vi "DIAdem Init.vi"(8 "error in (no error)":errorcluster, 10 "Startup DIAdem? (f)":bool) -> (0 "error out":errorcluster, 2 "Queues":T1, 3 "DIAdem Reference":T2)   [LabVIEW 2011]
uses:
  <vilib>/ExportToExcel/DIAdem Reference.ctl
  DIAdem Queues.ctl
  DIAdem Daemon Queue.ctl
  DIAdem Daemon Script Type.ctl
  Datasheet/Datasheet Inputs.ctl
  www/cgi-bin/_cgi-lib/TDM_INDEX Record.ctl
  Datasheet/Datasheet Generator Settings.ctl
  www/cgi-bin/runtest/runtest Queue.ctl
  www/tests/Test Output.ctl
  database/Fields/Field Record.ctl
  database/Fields/Field DataTypes.ctl
  database/Fields/Field NextItem.ctl
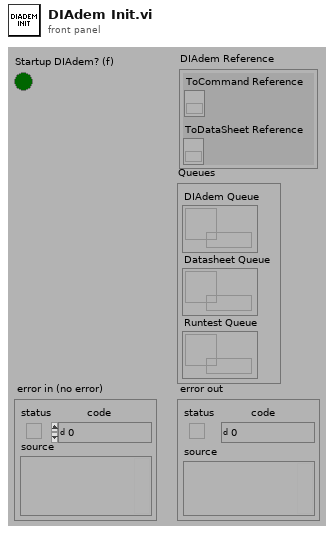
[diagram p1: front panel]
types:
  T1 = typedef "DIAdem Queues.ctl" = cluster{"DIAdem Queue":refnum<queue>, "Datasheet Queue":refnum<queue>, "Runtest Queue":refnum<queue>}
  T2 = typedef "DIAdem Reference.ctl" = cluster{"ToCommand Reference":refnum<k7>, "ToDataSheet Reference":refnum<k7>}
  T3 = typedef "runtest Queue.ctl" = cluster{"Test Output":T4, "Overwrite Existing?":bool, "Print?":bool, "sTestId":string, "Test Station IP (\"\")":string, "sxUsername (\"\")":string, "sDatasheetsCSV (\"\")":string, "Fields":T5[]}
  T4 = typedef "Test Output.ctl" = cluster{"Status":string, "Message":string, "Results":string, "Abort All":bool, "Save Results?":bool, "Timing Metrics":string}
  T5 = typedef "Field Record.ctl" = cluster{"ixField":i32, "iSequenceOrder":i32, "sxFieldId":string, "sxSequenceId":string, "sDisplayName":string, "sValue":string, "sUnits":string, "nDataType":T6, "nNextItem":T7, "fSystem":bool, "fSystemValue":bool, "fRequired":bool, "fSetAtTest":bool, "fTestField":bool, "fDeleted":bool, "fIndexed":bool, "fFreeList":bool}
  T6 = typedef "Field DataTypes.ctl" = enum32{"text", "numeric", "list", "timestamp", "boolean"}
  T7 = typedef "Field NextItem.ctl" = enum32{"Reset", "Retain", "Auto-Increment"}
  T8 = typedef "DATASHEET INPUTS.ctl" = cluster{"Items":T9[], "Templates":string[], "Generator Settings":T10, "Response Queue Name":string}
  T9 = typedef "TDM_INDEX Record.ctl" = cluster{"Model Number":string, "SN for sort":i32, "Test Type":string, "Test Run":string, "Serial Number":string, "Start Timestamp":timestamp, "Data File":path, "Result Columns":string[]}
  T10 = typedef "DATASHEET Generator Settings.ctl" = cluster{"Wait? (t)":bool, "ClientPrint? (f)":bool, "Client (\"\")":string, "joinPDF":bool, "Sort Method":enum16{"Item", "Template", "No Sort"}, "Export Row (-1=all)":i32, "Preview":bool, "Estimate Time":bool, "username":string, "jobid":string}
  T11 = typedef "DIAdem Daemon Queue.ctl" = cluster{"Report Template TDM":path, "Report Processor VBS":path, "Report Path PDF":path, "Report Script Params":string, "Username":string, "Script Type":T12, "Report Query Params":string, "Client Machine":string, "Print on Client?":bool, "Response Queue Name":string, "Script Variables":string[], "Start Request Time":timestamp, "Wait?":bool}
  T12 = typedef "DIAdem Daemon Script Type.ctl" = enum16{"Report", "Query", "Script", "Datasheet", "Append", "Restart", "Stop"}
  T13 = enum32{"invalid app kind", "Development System", "Run Time System", "Student Edition", "Embedded LabVIEW", "Evaluation", "Custom"}
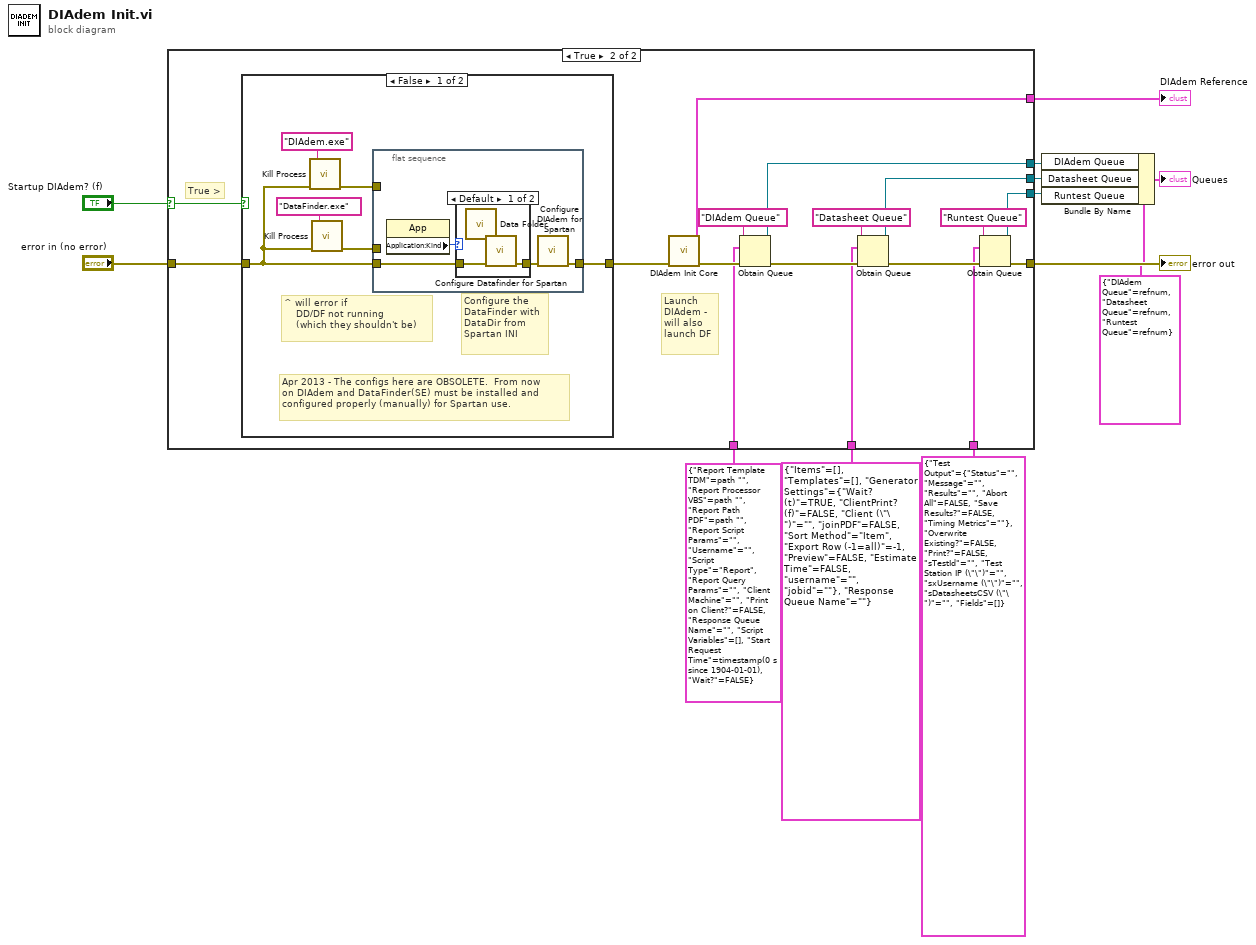
[diagram p0: block diagram]
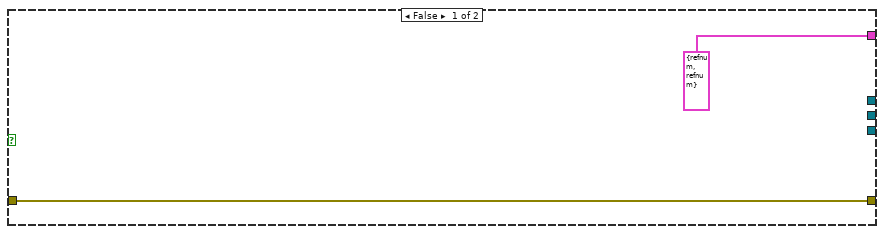
[diagram p2: hidden frame]
diagram:
  n1 = case shown="True" "Startup DIAdem? (f)" {
    selector: "Startup DIAdem? (f)" -> [_ w15]
    tunnel: "error in (no error)" -> [w14 w26]
    tunnel: [w14 w20] -> w11
    tunnel: [T2 {"ToCommand Reference"=refnum, "ToDataSheet Reference"=refnum} ("DIAdem Reference") w31] -> w9
    tunnel: [_ w28] -> w7
    tunnel: T11 {"Report Template TDM"=path "", "Report Processor VBS"=path "", "Report Path PDF"=path "", "Report Script Params"="", "Username"="", "Script Type"=enum."Report", "Report Query Params"="", "Client Machine"="", "Print on Client?"=FALSE, "Response Queue Name"="", "Script Variables"=[], "Start Request Time"=timestamp(0 s since 1904-01-01), "Wait?"=FALSE} ("DD_Report") -> [_ w25]
    tunnel: [_ w19] -> w6
    tunnel: [_ w18] -> w5
    tunnel: T8 {"Items"=[], "Templates"=[], "Generator Settings"={"Wait? (t)"=TRUE, "ClientPrint? (f)"=FALSE, "Client (\"\")"="", "joinPDF"=FALSE, "Sort Method"=enum."Item", "Export Row (-1=all)"=-1, "Preview"=FALSE, "Estimate Time"=FALSE, "username"="", "jobid"=""}, "Response Queue Name"=""} ("Datasheet Inputs") -> [_ w17]
    tunnel: T3 {"Test Output"={"Status"="", "Message"="", "Results"="", "Abort All"=FALSE, "Save Results?"=FALSE, "Timing Metrics"=""}, "Overwrite Existing?"=FALSE, "Print?"=FALSE, "sTestId"="", "Test Station IP (\"\")"="", "sxUsername (\"\")"="", "sDatasheetsCSV (\"\")"="", "Fields"=[]} ("INPUTS") -> [_ w16]
    frame False {
    }
    frame True {
      # "True >"
      # "Launch\nDIAdem -\nwill also\nlaunch DF"
      n2 = case shown="False" w15 {
        tunnel: [w36 w46] -> w27
        tunnel: w26 -> [w33 w46]
        frame False {
          # "Apr 2013 - The configs here are OBSOLETE.  From now\non DIAdem and DataFinder(SE) must be installed and\nconfigured properly (manually) for Spartan use."
          # "Configure the\nDataFinder with\nDataDir from\nSpartan INI"
          # "^ will error if\n    DD/DF not running\n    (which they shouldn't be)"
          n3 = call "Kill Process.vi"("error in (no error)"=w33, "Name of Process to kill (\"\")"="DIAdem.exe" ("Name of Process to kill (\"\")")) -> ("error out"=w32:errorcluster)  [unwired: 5 out]
          n4 = call "Kill Process.vi"("error in (no error)"=w33, "Name of Process to kill (\"\")"="DataFinder.exe" ("Name of Process to kill (\"\")")) -> ("error out"=w35:errorcluster)  [unwired: 5 out]
          n5 = flat-sequence {
            tunnel: w33 -> [w41]
            tunnel: [w39] -> w36
            tunnel: w35 -> [_]
            tunnel: w32 -> [_]
            frame #0 {
              n6 = property class="App"() -> ("Application:Kind"=w40:T13)  [unwired: 2 in, 2 out]
              n7 = case shown="Default" w40 {
                tunnel: w41 -> [w44 w45]
                tunnel: [w42 w45] -> w38
                frame Default {
                  n8 = call "Data Folder.vi"() -> ("Data Folder"=w43:path)  [unwired: 3 in]
                  n9 = call "Configure Datafinder for Spartan.vi"("error in (no error)"=w44, "Data Path"=w43) -> ("error out"=w42:errorcluster)  [unwired: 9 in]
                }
                frame "Development System" {
                }
              }
              n10 = call "Configure DIAdem for Spartan.vi"("error in (no error)"=w38) -> ("error out"=w39:errorcluster)  [unwired: 10 in]
            }
          }
        }
        frame True {
          # "This case should run - the FALSE case\nis there for reference."
        }
      }
      n11 = call "DIAdem Init Core.vi"("error in"=w27) -> ("error out"=w29:errorcluster, "DIAdem Reference"=w31:T2)  [unwired: 9 out]
      n12 = Obtain Queue(name (unnamed)="DIAdem Queue", element data type=w25, error in (no error)=w29) -> (queue out=w28:refnum<queue>, error out=w22:errorcluster)  [unwired: 2 in, 1 out]
      n13 = Obtain Queue(name (unnamed)="Datasheet Queue", element data type=w17, error in (no error)=w22) -> (queue out=w19:refnum<queue>, error out=w21:errorcluster)  [unwired: 2 in, 1 out]
      n14 = Obtain Queue(name (unnamed)="Runtest Queue", element data type=w16, error in (no error)=w21) -> (queue out=w18:refnum<queue>, error out=w20:errorcluster)  [unwired: 2 in, 1 out]
    }
  }
  "error out" <- w11
  "DIAdem Reference" <- w9
  n15 = Bundle By Name(cluster=T1 {"DIAdem Queue"=refnum, "Datasheet Queue"=refnum, "Runtest Queue"=refnum} ("Queues"), "DIAdem Queue"=w7, "Datasheet Queue"=w6, "Runtest Queue"=w5) -> (→"Queues":T1)
